vi "Increment halfmove counter.vi"(8 "error in (no error)":errorcluster, 11 "Position in":refnum<class "Position.lvclass">) -> (0 "error out":errorcluster, 3 "Position out":refnum<class "Position.lvclass">)   [LabVIEW 2015, in "Chesslib.lvlib" / "Position.lvclass"]
uses:
  Position.lvclass
  Position.lvclass/Position.ctl
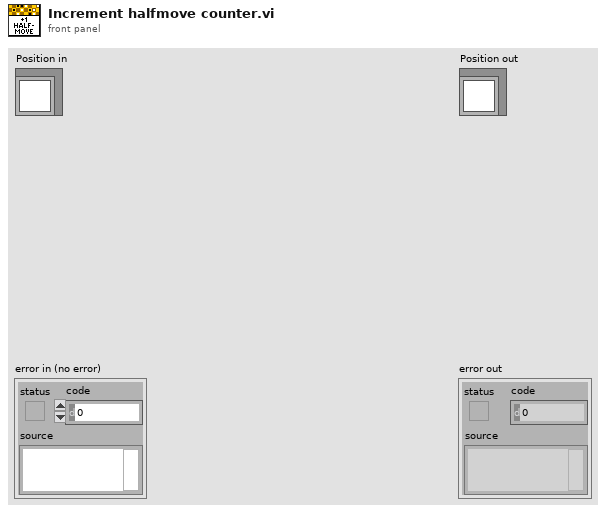
[diagram p1: front panel]
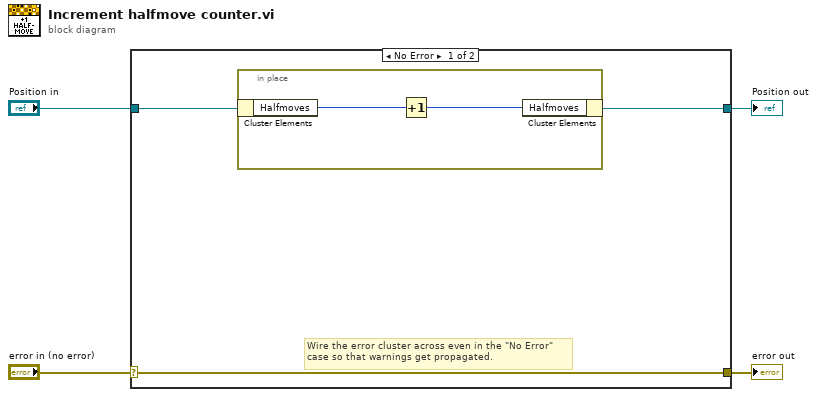
[diagram p0: block diagram]
diagram:
  n1 = case shown="No Error" "error in (no error)" {
    selector: "error in (no error)" -> [w7 w11]
    tunnel: [w7 w11] -> w3
    tunnel: [w5 w10] -> w1
    tunnel: "Position in" -> [w6 w10]
    frame No Error {
      # "Wire the error cluster across even in the \"No Error\"\ncase so that warnings get propagated."
      n2 = in-place {
        n3 = in-place-cluster #1(w6) -> ("Halfmoves"=w9:u8)
        n4 = Increment(x=w9) -> (x+1=w8:u8)
        n5 = in-place-cluster #1("Halfmoves"=w8) -> (w5:refnum<class "Position.lvclass">)
      }
    }
    frame Error {
    }
  }
  "error out" <- w3
  "Position out" <- w1
